vi "LVClass_Pupil ctor from Legendre pupil.vi"(0 "Pupil.lvclass":refnum<class "Pupil.lvclass">, 5 "Dimensions_um":T2={"Size"={"X"=1, "Y"=2}, "Step"={"X"=3.0, "Y"=4.0}}, 7 "center":T1, 9 "halfsize_rectangle":T1, 11 "error constant":errorcluster) -> (4 "Pupil (new)":refnum<class "Pupil.lvclass">, 15 "error IO":errorcluster)   [LabVIEW 2020, in "Pupil.lvclass"]
doc: "Rectangular Pupil constructor from dimensions, steps and rectangle shape.\n\n--------------------------------------------------------------------------------\n\n<B>PupilIn </B> : Constant Pointer to Pupil object.\n<B>PupilOut </B> : Constant Pointer to Pupil object.\n<B>step </B> : Step x and y between the subpupils (um).\n<B>dimensions </B> : Pupil array dimensions (width, height).\n<B>center </B> : Center of the rectangle shape (um).\n<B>rectangle_size </B> : Shape (width, height) of the rectangle (um).\n<B>ErrorIn </B> : Error\n<B>ErrorOut </B> : Error\n\n--------------------------------------------------------------------------------"
uses:
  Pupil.lvclass
  Controls/General dimensions definition.ctl
  Controls/Point2D.ctl
  Controls/Point2Df.ctl
  Controls/Handle creation.ctl
  Pupil.lvclass/Pupil.ctl
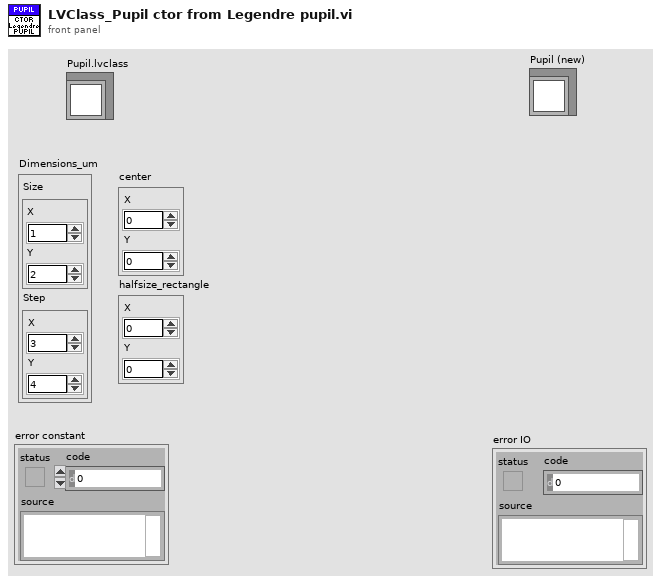
[diagram p1: front panel]
types:
  T1 = typedef "Point2Df.ctl" = cluster{"X":sgl, "Y":sgl}
  T2 = typedef "General dimensions definition.ctl" = cluster{"Size":T3, "Step":T1}
  T3 = typedef "Point2D.ctl" = cluster{"X":u32, "Y":u32}
  T4 = typedef "Handle creation.ctl" = enum16{"By ctor", "By write function"}
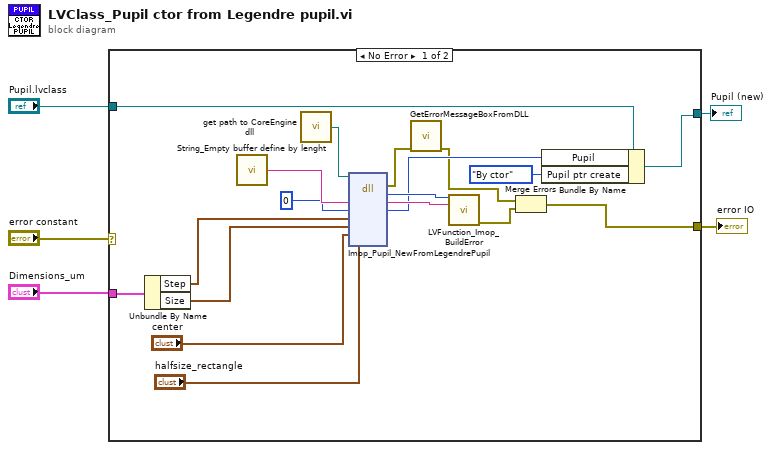
[diagram p0: block diagram]
diagram:
  n1 = case shown="No Error" "error constant" {
    selector: "error constant" -> [_ w25]
    tunnel: [w6 w25] -> w4
    tunnel: [w16 w24] -> w2
    tunnel: "Pupil.lvclass" -> [w17 w24]
    tunnel: "Dimensions_um" -> [w13 _]
    frame No Error {
      n2 = Unbundle By Name(w13) -> ("Step"=w9:T1, "Size"=w12:T3)
      n3 = call "String_Empty buffer define by lenght.vi"() -> ("Empty buffer"=w23:string)  [unwired: 1 in]
      n4 = call "get path to CoreEngine dll.vi"() -> ("path to wavekit library"=w20:path)  [unwired: 14 in, 1 out]
      n5 = dll-call lib="D:/soft/HASO_v3/SVN_trunk/ImOpCoreEngine4_LV2011/DLLs/c_interface_vc100.dll" fn="Imop_Pupil_NewFromLegendrePupil"(path in=w20, "message"=w23, "Pupil"=0, "step"=w9, "sizePupil"=w12, "center"="center", "size2Rectangle"="halfsize_rectangle") -> (error out=w19:errorcluster, "return type"=w21:i32, "message"=w22:string, "Pupil"=w15:i64)  [unwired: 6 in, 1 out]
      n6 = call "GetErrorMessageBoxFromDLL.vi"("error IN"=w19) -> ("error OUT"=w8:errorcluster)  [unwired: 10 in]
      n7 = call "LVFunction_Imop_BuildError.vi"("code"=w21, "String to Prepend to source (\"\")"=w22) -> ("error out"=w7:errorcluster)  [unwired: 13 in]
      n8 = Merge Errors(w8, w7) -> (w6:errorcluster)
      n9 = Bundle By Name(cluster=w17, "Pupil"=w15, "Pupil ptr create"=Handle_creation."By ctor") -> (w16:refnum<class "Pupil.lvclass">)
    }
    frame Error {
    }
  }
  "error IO" <- w4
  "Pupil (new)" <- w2
